vi "Read Bottom Panel ref.vi"(8 "error in":errorcluster, 11 "Base Software in":refnum<class "Base Software.lvclass">) -> (0 "error out":errorcluster, 2 "Bottom Panel":refnum<vi>, 3 "Base Software out":refnum<class "Base Software.lvclass">)   [LabVIEW 2019, in "Base Software.lvlib" / "Main.lvlib" / "Base Software.lvclass"]
uses:
  Project/Base Software.lvclass
  Project/Base Software.lvclass/Base Software.ctl
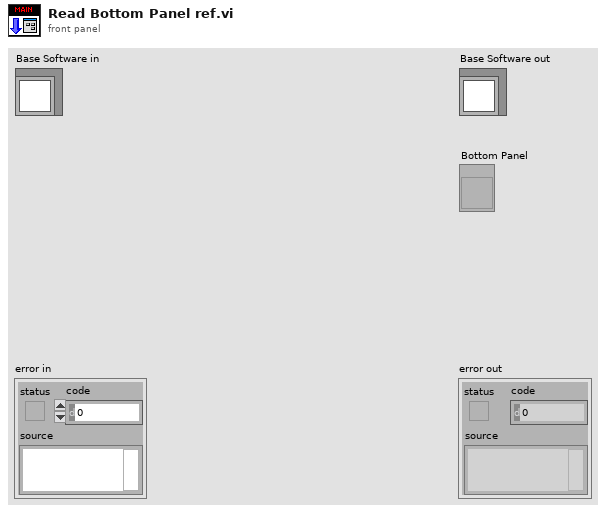
[diagram p1: front panel]
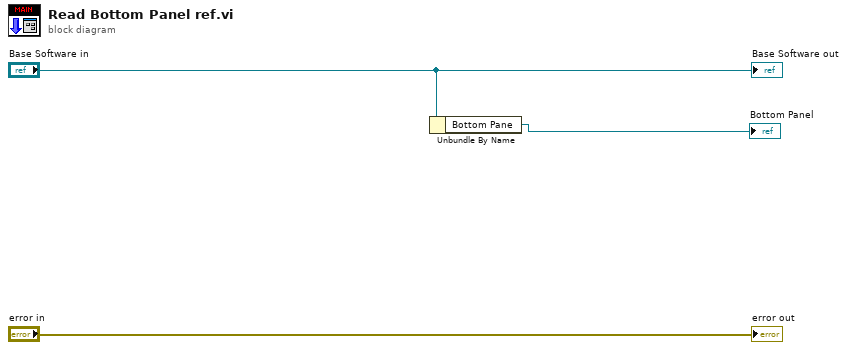
[diagram p0: block diagram]
diagram:
  n1 = Unbundle By Name("Base Software in") -> ("Bottom Pane"=→"Bottom Panel":refnum<vi>)
  "error out" <- "error in"
  "Base Software out" <- "Base Software in"
